vi "Application.vi"() -> ()   [LabVIEW 2021]
doc: "Application that demonstrates connecting to a DAQ device and activates the selected digital inputs and analog inputs. Stream the data from devices, logging the datapoints to CSV file and 2 plots."
uses:
  TypeDefs/TypeDef - Cluster of DAQiFi Device Properties.ctl
  TypeDefs/Enum - Connection Type.ctl
  <vilib>/Utility/file.llb/Write Delimited Spreadsheet (string).vi
  <vilib>/JDP Science/JDP Science Common Utilities/Timestamp/JDP Timestamp.lvlib
panel:
  in  "Data Logging Rate (Hz)":i32=10 min=1 max=1000 step=1
  in  "Start Logging":bool
  in  "Filepath to Save Data to (CSV)":path
  in  "Digital Channels":bool[](array[boolean])
  in  "Analog Channels":bool[](array[boolean])
  in  "Connect USB":bool
  out "Busy":u16(ring)
  out "Status":string
  in  "Connect WIFI":bool
  in  "Search USB":bool
  in  "Search WIFI":bool
  in  "DAQiFi Available USB Connections":i32(listbox)
  in  "DAQiFi Available Wireless Connections":i32(listbox)
  out "Digital Chart":T1(graph)
  out "Analog Chart":T2(graph)
  in  "stop":bool
  # "Enabled selected channels by left clicking the green boxes"
  # "0       1      2      3     4      5     6      7      8     9     10    11    12    13   14    15"
  # "0       1      2      3     4      5     6      7      8     9     10    11    12    13   14    15"
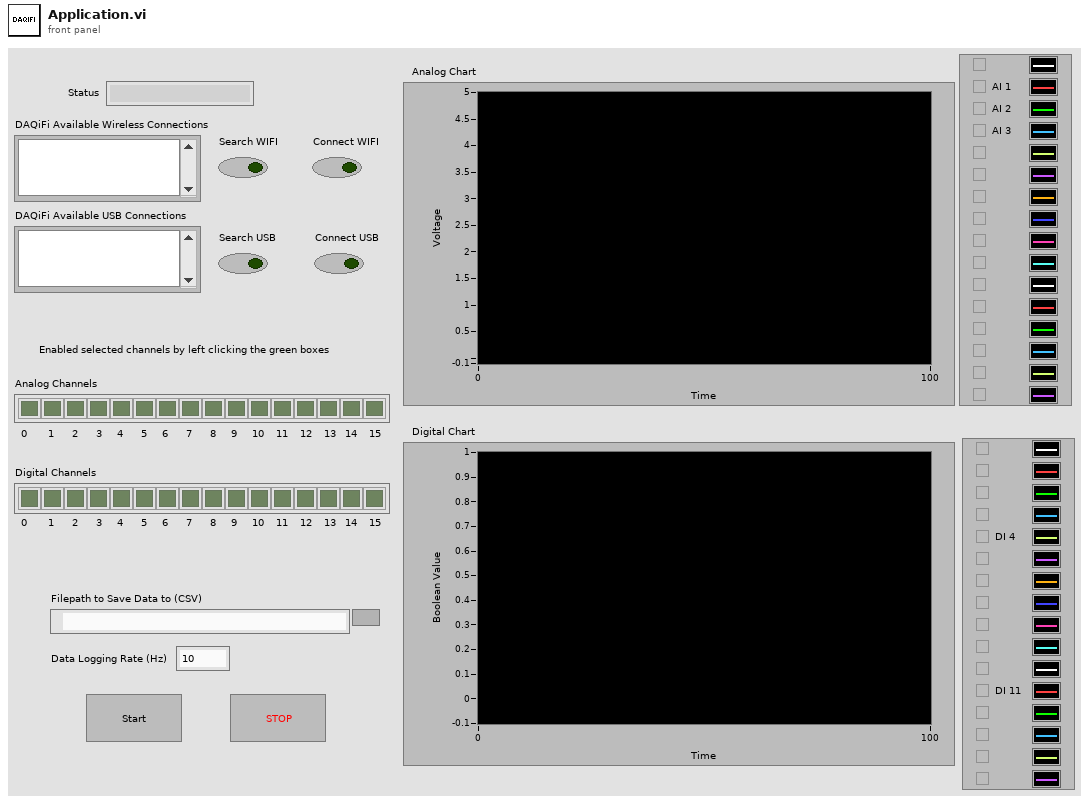
[diagram p1: front panel]
types:
  T1 = cluster{"[0]":dbl, "[1]":dbl, "[2]":dbl, "[3]":dbl, "[4]":dbl, "[5]":dbl, "[6]":dbl, "[7]":dbl, "[8]":dbl}
  T2 = cluster{"Array of Voltages (V)[0]":dbl, "Array of Voltages (V)[1]":dbl, "Array of Voltages (V)[2]":dbl, "Array of Voltages (V)[3]":dbl, "Array of Voltages (V)[4]":dbl, "Array of Voltages (V)[5]":dbl, "Array of Voltages (V)[6]":dbl, "Array of Voltages (V)[7]":dbl, "Array of Voltages (V)[8]":dbl}
  T3 = typedef "TypeDef - Cluster of DAQiFi Device Properties.ctl" = cluster{"IP Address":string, "MAC Address":string, "Serial Number":string, "Connection Type":T4, "Connected":bool, "TCP Network Connection":refnum<k5>, "USB Serial Connection":refnum<visa-resource-name>}
  T4 = typedef "Enum - Connection Type.ctl" = enum16{"USB", "TCP"}
  T5 = cluster{"Array of Voltages (V)[0]":dbl, "Array of Voltages (V)[1]":dbl, "Array of Voltages (V)[2]":dbl, "Array of Voltages (V)[3]":dbl, "Array of Voltages (V)[4]":dbl, "Array of Voltages (V)[5]":dbl, "Array of Voltages (V)[6]":dbl, "Array of Voltages (V)[7]":dbl, "Array of Voltages (V)[8]":dbl}[]
  T6 = enum8{"Enabled", "Disabled", "Disabled and Grayed Out"}
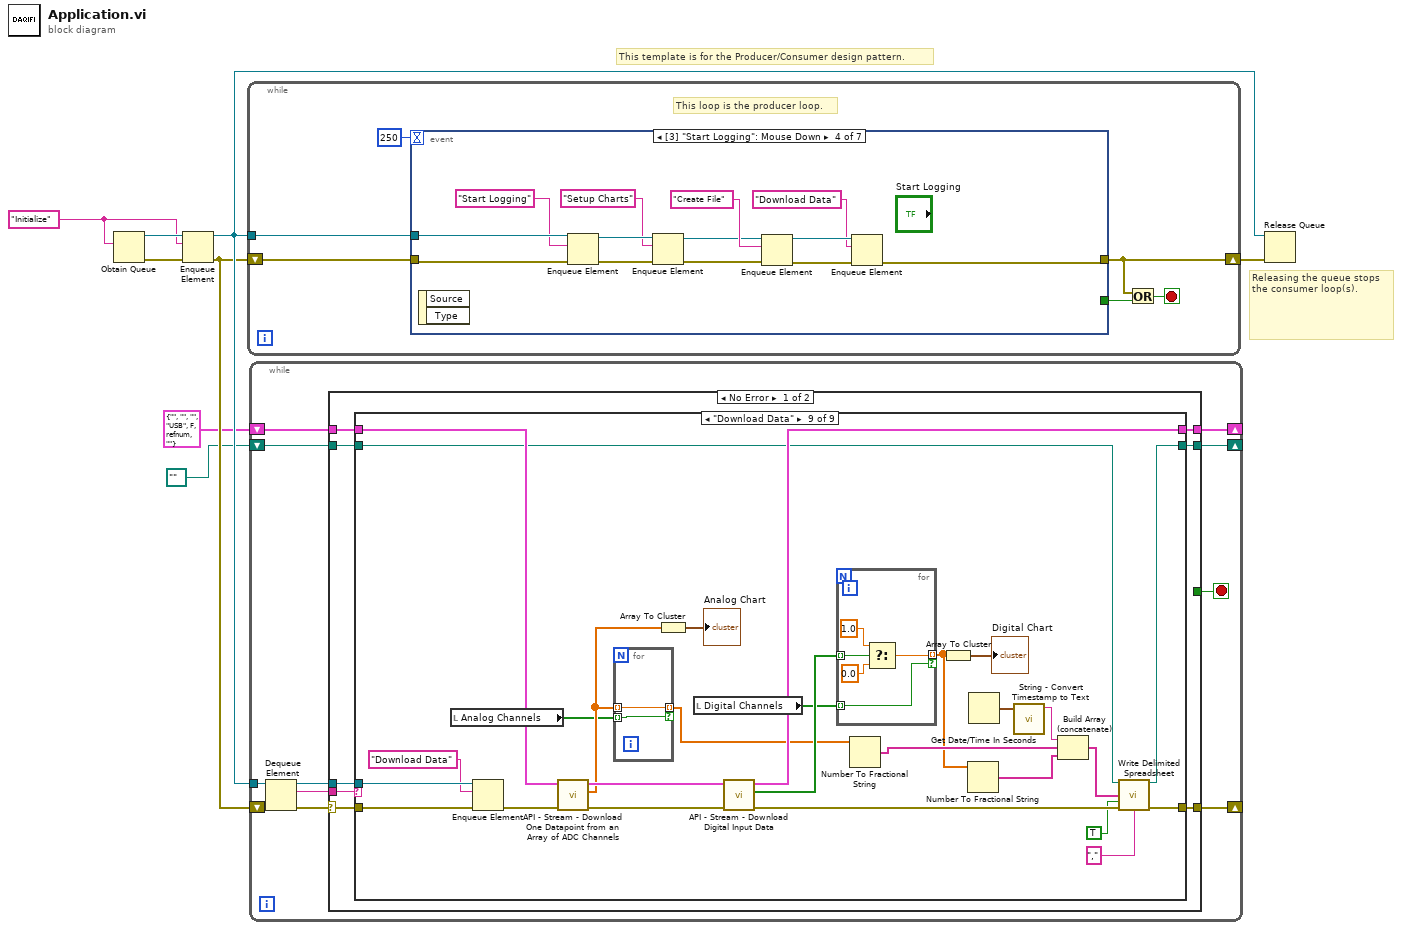
[diagram p0: block diagram]
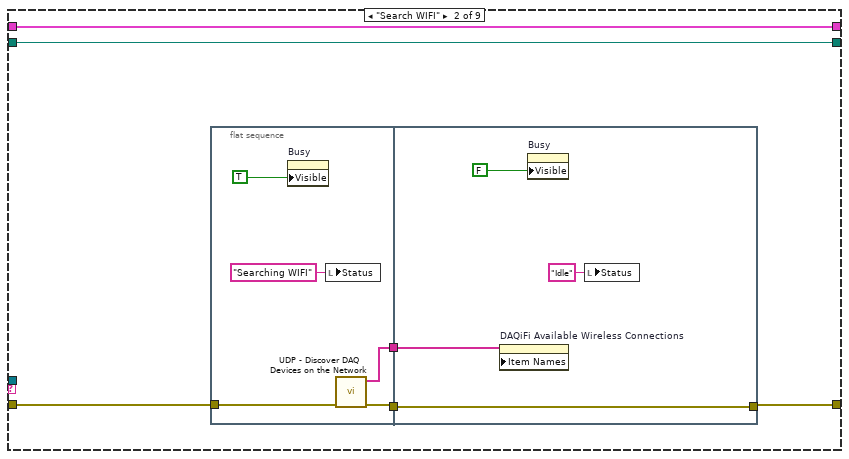
[diagram p3: hidden frame]
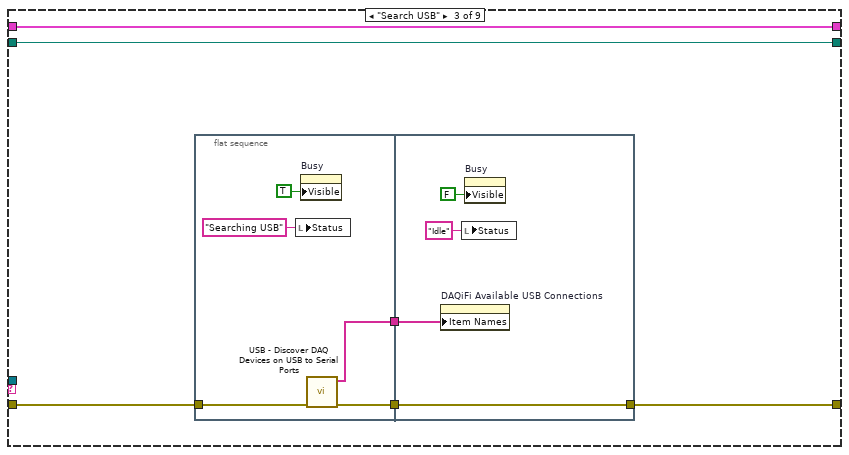
[diagram p4: hidden frame]
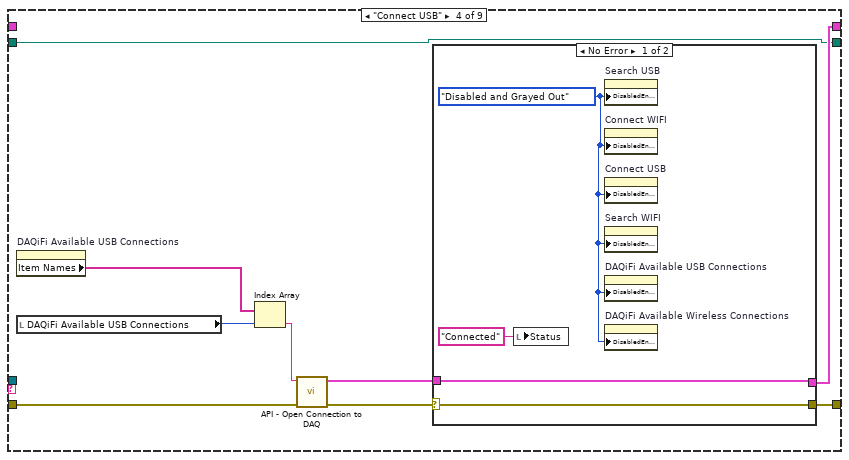
[diagram p5: hidden frame]
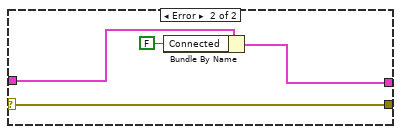
[diagram p6: hidden frame]
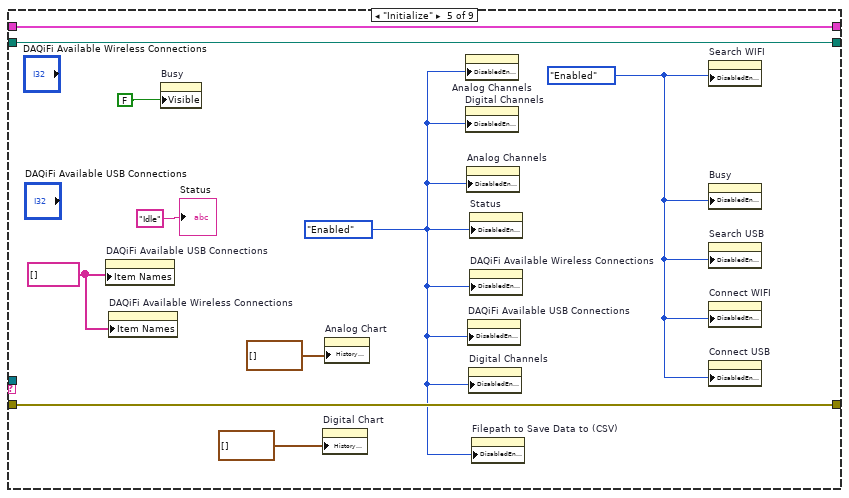
[diagram p7: hidden frame]
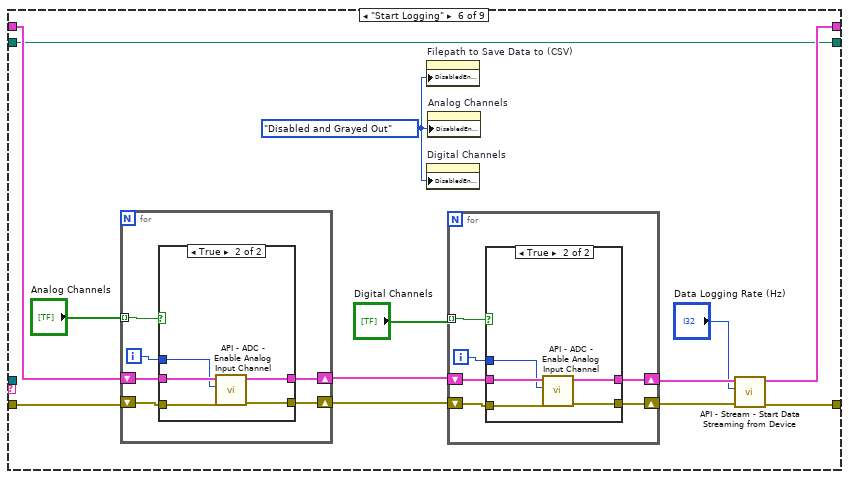
[diagram p8: hidden frame]
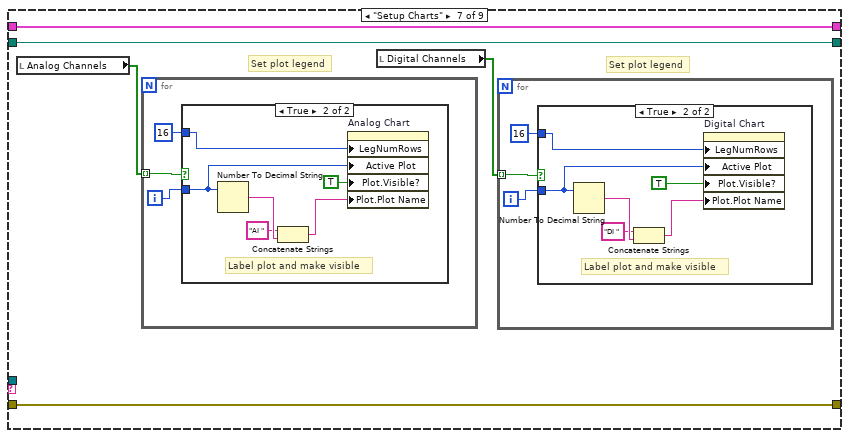
[diagram p11: hidden frame]
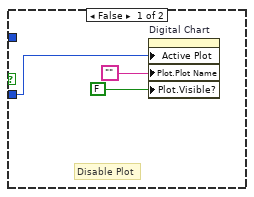
[diagram p12: hidden frame]
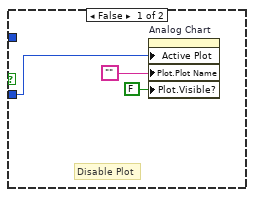
[diagram p13: hidden frame]
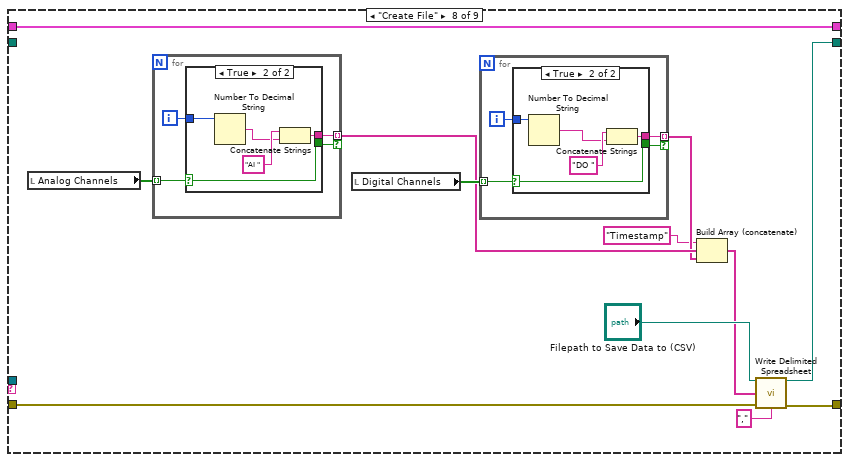
[diagram p14: hidden frame]
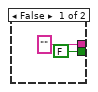
[diagram p15: hidden frame]
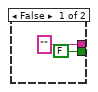
[diagram p16: hidden frame]
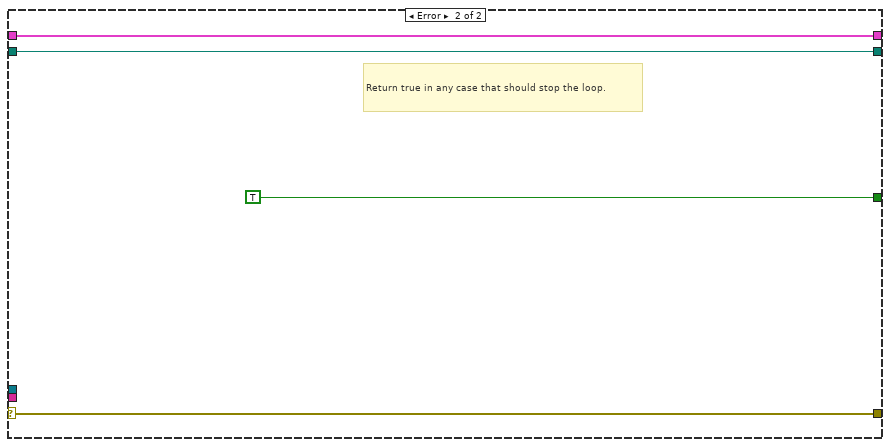
[diagram p17: hidden frame]
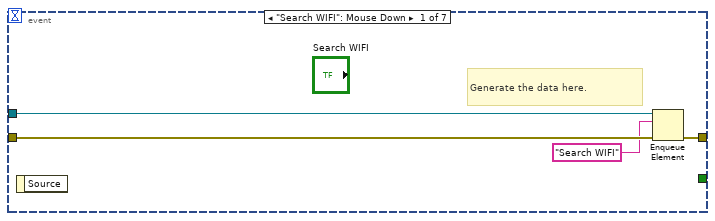
[diagram p18: hidden frame]
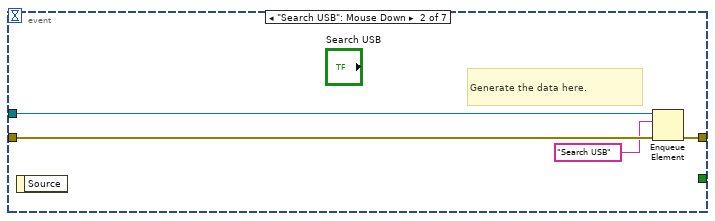
[diagram p19: hidden frame]
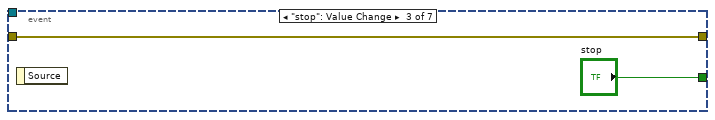
[diagram p20: hidden frame]
diagram:
  w4 = "Initialize"
  # "Releasing the queue stops the consumer loop(s)."
  # "This template is for the Producer/Consumer design pattern."
  n1 = Obtain Queue(element data type=w4) -> (queue out=w7:refnum<queue>, error out=w6:errorcluster)  [unwired: 4 in, 1 out]
  n2 = Enqueue Element(queue=w7, element=w4, error in (no error)=w6) -> (queue out=w5:refnum<queue>, error out=w3:errorcluster)  [unwired: 1 in, 1 out]
  n3 = while {
    shift-right: [w10] -> w8
    shift-left: w3 -> [w13]
    tunnel: w5 -> [w14]
    stop <- w11 stop-if-true
    # "This loop is the producer loop."
    n4 = event shown="[3] \"Start Logging\": Mouse Down" {
      selector: _ -> [_ _ _ _ _ _ _]
      dyn-events: _ -> [_ _ _ _ _ _ _]
      timeout: 250 -> [_ _ _ _ _ _ _]
      tunnel: w14 -> [w18 w22 _ w37 _ w47 w51]
      tunnel: w13 -> [w17 w21 w23 w36 _ w46 w50]
      tunnel: [w16 w20 w23 w33 _ w45 w49] -> w10
      tunnel: [_ _ "stop" _ _ _ _] -> w12
      event "Search WIFI": Mouse Down {
        # "Generate the data here."
        n5 = event-data() -> ()  [unwired: 1 in, 1 out]
        n6 = Enqueue Element(queue=w18, element="Search WIFI", error in (no error)=w17) -> (error out=w16:errorcluster)  [unwired: 1 in, 2 out]
      }
      event "Search USB": Mouse Down {
        # "Generate the data here."
        n7 = event-data() -> ()  [unwired: 1 in, 1 out]
        n8 = Enqueue Element(queue=w22, element="Search USB", error in (no error)=w21) -> (error out=w20:errorcluster)  [unwired: 1 in, 2 out]
      }
      event "stop": Value Change {
        n9 = event-data() -> ()  [unwired: 1 in, 1 out]
      }
      event "Start Logging": Mouse Down {
        n10 = event-data() -> ()  [unwired: 1 in, 2 out]
        n11 = Enqueue Element(queue=w37, element="Start Logging", error in (no error)=w36) -> (queue out=w26:refnum<queue>, error out=w29:errorcluster)  [unwired: 1 in, 1 out]
        n12 = Enqueue Element(queue=w26, element="Setup Charts", error in (no error)=w29) -> (queue out=w27:refnum<queue>, error out=w28:errorcluster)  [unwired: 1 in, 1 out]
        n13 = Enqueue Element(queue=w27, element="Create File", error in (no error)=w28) -> (queue out=w32:refnum<queue>, error out=w34:errorcluster)  [unwired: 1 in, 1 out]
        n14 = Enqueue Element(queue=w32, element="Download Data", error in (no error)=w34) -> (error out=w33:errorcluster)  [unwired: 1 in, 2 out]
      }
      event Timeout {
        n15 = event-data() -> ()  [unwired: 1 in, 2 out]
        n16 = local read "Busy"() -> (w43:u16)
        n17 = Increment(x=w43) -> (x+1=w39:u16)
        n18 = Greater?(x=w39, y=u16 6) -> (0:w41:bool)
        n19 = Select(t=u16 0, s=w41, f=w39) -> (s? t:f=→"Busy":u16)
      }
      event "Connect USB": Value Change {
        n20 = event-data() -> ()  [unwired: 1 in, 2 out]
        n21 = Enqueue Element(queue=w47, element="Connect USB", error in (no error)=w46) -> (error out=w45:errorcluster)  [unwired: 1 in, 2 out]
      }
      event "Connect WIFI": Value Change {
        n22 = event-data() -> ()  [unwired: 1 in, 2 out]
        n23 = Enqueue Element(queue=w51, element="Connect WIFI", error in (no error)=w50) -> (error out=w49:errorcluster)  [unwired: 1 in, 2 out]
      }
    }
    n24 = Or(x=w10, y=w12) -> (x .or. y?=w11:bool)
  }
  n25 = while {
    tunnel: w5 -> [w62]
    shift-right: [w58] -> _
    shift-left: w3 -> [w57]
    shift-right: [w56] -> _
    shift-left: T3 {"IP Address"="", "MAC Address"="", "Serial Number"="", "Connection Type"=enum."USB", "Connected"=FALSE, "TCP Network Connection"=refnum, "USB Serial Connection"=""} ("DAQiFi Device Properties") -> [w55]
    shift-right: [w54] -> _
    shift-left: path "" ("new file path (Not A Path if cancelled)") -> [w53]
    stop <- w59 stop-if-true
    n26 = Dequeue Element(queue=w62, error in (no error)=w57) -> (queue out=w52:refnum<queue>, element=w60:string, error out=w61:errorcluster)  [unwired: 1 in, 1 out]
    n27 = case shown="No Error" w61 {
      selector: w61 -> [w69 w268]
      tunnel: w60 -> [w70 _]
      tunnel: [_ TRUE] -> w59
      tunnel: [w68 w268] -> w58
      tunnel: [w67 w269] -> w56
      tunnel: w55 -> [w66 w269]
      tunnel: [w65 w267] -> w54
      tunnel: w53 -> [w64 w267]
      tunnel: w52 -> [w63 _]
      frame No Error {
        n28 = case shown="\"Download Data\"" w70 {
          tunnel: w69 -> [w73 w77 w93 w110 w129 w141 w174 w209 w258]
          tunnel: [w73 w75 w92 w105 w129 w135 w174 w208 w246] -> w68
          tunnel: [w72 w78 w94 w106 w128 w134 w173 w210 w252] -> w67
          tunnel: w66 -> [w72 w78 w94 _ w128 w142 w173 w210 w255]
          tunnel: [w71 w74 w89 w104 w123 w131 w172 w200 w244] -> w65
          tunnel: w64 -> [w71 w74 w89 w104 w123 w131 w172 _ w245]
          tunnel: w63 -> [_ _ _ _ _ _ _ _ w259]
          frame "False", Default {
          }
          frame "Search WIFI" {
            n29 = flat-sequence {
              tunnel: [w84] -> w79
              tunnel: w77 -> [w81]
              tunnel: [w80] -> w76
              tunnel: w79 -> [w88]
              tunnel: [w85] -> w75
              tunnel: w76 -> [w85]
              frame #0 {
                n30 = property on="Busy" class="Ring (strict)"("Visible"=TRUE) -> ()  [unwired: 2 in, 2 out]
                n31 = local write "Status"("Searching WIFI" ("Status")) -> ()
                n32 = call "UDP - Discover DAQ Devices on the Network.vi"("error in"=w81) -> ("Error out"=w80:errorcluster, "List of IPs"=w84:string[])  [unwired: 8 in, 1 out]
              }
              frame #1 {
                n33 = property on="DAQiFi Available Wireless Connections" class="LstBox (strict)"("Item Names"=w88) -> ()  [unwired: 2 in, 2 out]
                n34 = property on="Busy" class="Ring (strict)"("Visible"=FALSE) -> ()  [unwired: 2 in, 2 out]
                n35 = local write "Status"("Idle" ("Status")) -> ()
              }
            }
          }
          frame "Search USB" {
            n36 = flat-sequence {
              tunnel: w93 -> [w99]
              tunnel: [w98] -> w91
              tunnel: [w95] -> w90
              tunnel: [w103] -> w92
              tunnel: w91 -> [w103]
              tunnel: w90 -> [w100]
              frame #0 {
                n37 = local write "Status"("Searching USB" ("Status")) -> ()
                n38 = property on="Busy" class="Ring (strict)"("Visible"=TRUE) -> ()  [unwired: 2 in, 2 out]
                n39 = call "USB - Discover DAQ Devices on USB to Serial Ports.vi"("error in"=w99) -> ("error out"=w98:errorcluster, "List of DAQiFi COM Ports"=w95:string[])  [unwired: 8 in, 1 out]
              }
              frame #1 {
                n40 = property on="DAQiFi Available USB Connections" class="LstBox (strict)"("Item Names"=w100) -> ()  [unwired: 2 in, 2 out]
                n41 = local write "Status"("Idle" ("Status")) -> ()
                n42 = property on="Busy" class="Ring (strict)"("Visible"=FALSE) -> ()  [unwired: 2 in, 2 out]
              }
            }
          }
          frame "Connect USB" {
            n43 = property on="DAQiFi Available USB Connections" class="LstBox (strict)"() -> ("Item Names"=w112:string[])  [unwired: 2 in, 2 out]
            n44 = local read "DAQiFi Available USB Connections"() -> (w109:i32)
            n45 = Index Array(array=w112, index=w109) -> (element=w111:string)
            n46 = call "API - Open Connection to DAQ.vi"("error in"=w110, "DAQ Address (IP or COM)"=w111) -> ("error out"=w108:errorcluster, "DAQiFi Device Properties"=w107:T3)  [unwired: 8 in]
            n47 = case shown="No Error" w108 {
              selector: w108 -> [w116 w117]
              tunnel: w107 -> [w115 w120]
              tunnel: [w115 w118] -> w106
              tunnel: [w116 w117] -> w105
              frame No Error {
                w114 = T6."Disabled and Grayed Out" ("Disabled")
                n48 = local write "Status"("Connected" ("Status")) -> ()
                n49 = property on="Search USB" class="Bool (strict)"("DisabledEnum"=w114) -> ()  [unwired: 2 in, 2 out]
                n50 = property on="Connect WIFI" class="Bool (strict)"("DisabledEnum"=w114) -> ()  [unwired: 2 in, 2 out]
                n51 = property on="Connect USB" class="Bool (strict)"("DisabledEnum"=w114) -> ()  [unwired: 2 in, 2 out]
                n52 = property on="Search WIFI" class="Bool (strict)"("DisabledEnum"=w114) -> ()  [unwired: 2 in, 2 out]
                n53 = property on="DAQiFi Available USB Connections" class="LstBox (strict)"("DisabledEnum"=w114) -> ()  [unwired: 2 in, 2 out]
                n54 = property on="DAQiFi Available Wireless Connections" class="LstBox (strict)"("DisabledEnum"=w114) -> ()  [unwired: 2 in, 2 out]
              }
              frame Error {
                n55 = Bundle By Name(cluster=w120, "Connected"=FALSE) -> (w118:T3)
              }
            }
          }
          frame "Initialize" {
            w124 = T6."Enabled" ("Disabled")
            w125 = T6."Enabled" ("Disabled")
            w126 = string[] [] ("Item Names")
            n56 = property on="DAQiFi Available USB Connections" class="LstBox (strict)"("Item Names"=w126) -> ()  [unwired: 2 in, 2 out]
            n57 = property on="DAQiFi Available Wireless Connections" class="LstBox (strict)"("Item Names"=w126) -> ()  [unwired: 2 in, 2 out]
            n58 = property on="Busy" class="Ring (strict)"("Visible"=FALSE) -> ()  [unwired: 2 in, 2 out]
            n59 = property on="Digital Chart" class="WFChart (strict)"("History Data"=T5 []) -> ()  [unwired: 2 in, 2 out]
            n60 = property on="Analog Chart" class="WFChart (strict)"("History Data"=T5 []) -> ()  [unwired: 2 in, 2 out]
            n61 = property on="Analog Channels" class="Arr (strict)"("DisabledEnum"=w124) -> ()  [unwired: 2 in, 2 out]
            n62 = property on="Digital Channels" class="Arr (strict)"("DisabledEnum"=w124) -> ()  [unwired: 2 in, 2 out]
            n63 = property on="Analog Channels" class="Arr (strict)"("DisabledEnum"=w124) -> ()  [unwired: 2 in, 2 out]
            n64 = property on="DAQiFi Available USB Connections" class="LstBox (strict)"("DisabledEnum"=w124) -> ()  [unwired: 2 in, 2 out]
            n65 = property on="Digital Channels" class="Arr (strict)"("DisabledEnum"=w124) -> ()  [unwired: 2 in, 2 out]
            n66 = property on="Status" class="Str"("DisabledEnum"=w124) -> ()  [unwired: 2 in, 2 out]
            n67 = property on="DAQiFi Available Wireless Connections" class="LstBox (strict)"("DisabledEnum"=w124) -> ()  [unwired: 2 in, 2 out]
            n68 = property on="Filepath to Save Data to (CSV)" class="Path"("DisabledEnum"=w124) -> ()  [unwired: 2 in, 2 out]
            n69 = property on="Search WIFI" class="Bool (strict)"("DisabledEnum"=w125) -> ()  [unwired: 2 in, 2 out]
            n70 = property on="Busy" class="Ring (strict)"("DisabledEnum"=w125) -> ()  [unwired: 2 in, 2 out]
            n71 = property on="Search USB" class="Bool (strict)"("DisabledEnum"=w125) -> ()  [unwired: 2 in, 2 out]
            n72 = property on="Connect WIFI" class="Bool (strict)"("DisabledEnum"=w125) -> ()  [unwired: 2 in, 2 out]
            n73 = property on="Connect USB" class="Bool (strict)"("DisabledEnum"=w125) -> ()  [unwired: 2 in, 2 out]
            "Status" <- "Idle" ("Status")
          }
          frame "Start Logging" {
            w132 = T6."Disabled and Grayed Out" ("Disabled")
            n74 = for {
              tunnel: "Analog Channels" -> [w161] mode=indexing
              shift-right: [w158] -> w139
              shift-left: w142 -> [w162]
              shift-right: [w159] -> w138
              shift-left: w141 -> [w160]
              i -> [w157]
              n75 = case shown="True" w161 {
                tunnel: w162 -> [w164 w169]
                tunnel: w160 -> [w163 w168]
                tunnel: [w163 w167] -> w159
                tunnel: [w164 w166] -> w158
                tunnel: w157 -> [_ w165]
                frame False {
                }
                frame True {
                  n76 = call "API - ADC - Enable Analog Input Channel.vi"("error in (no error)"=w168, "Analog Input Channel Number"=w165, "DAQiFi Device Properties In"=w169) -> ("error out"=w167:errorcluster, "DAQiFi Device Properties Out"=w166:T3)  [unwired: 7 in]
                }
              }
            }
            n77 = property on="Filepath to Save Data to (CSV)" class="Path"("DisabledEnum"=w132) -> ()  [unwired: 2 in, 2 out]
            n78 = property on="Digital Channels" class="Arr (strict)"("DisabledEnum"=w132) -> ()  [unwired: 2 in, 2 out]
            n79 = property on="Analog Channels" class="Arr (strict)"("DisabledEnum"=w132) -> ()  [unwired: 2 in, 2 out]
            n80 = for {
              tunnel: "Digital Channels" -> [w148] mode=indexing
              shift-right: [w145] -> w136
              shift-left: w139 -> [w149]
              shift-right: [w146] -> w137
              shift-left: w138 -> [w147]
              i -> [w144]
              n81 = case shown="True" w148 {
                tunnel: w149 -> [w151 w156]
                tunnel: w147 -> [w150 w155]
                tunnel: [w150 w154] -> w146
                tunnel: [w151 w153] -> w145
                tunnel: w144 -> [_ w152]
                frame False {
                }
                frame True {
                  n82 = call "API - ADC - Enable Analog Input Channel.vi"("error in (no error)"=w155, "Analog Input Channel Number"=w152, "DAQiFi Device Properties In"=w156) -> ("error out"=w154:errorcluster, "DAQiFi Device Properties Out"=w153:T3)  [unwired: 7 in]
                }
              }
            }
            n83 = call "API - Stream - Start Data Streaming from Device.vi"("error in"=w137, "Streaming Rate (Hz)"="Data Logging Rate (Hz)", "DAQiFi Device Properties In"=w136) -> ("error out"=w135:errorcluster, "DAQiFi Device Properties Out"=w134:T3)  [unwired: 7 in]
          }
          frame "Setup Charts" {
            # "Set plot legend"
            # "Set plot legend"
            n84 = local read "Analog Channels"() -> (w171:bool[])
            n85 = for {
              tunnel: w171 -> [w189] mode=indexing
              i -> [w188]
              n86 = case shown="True" w189 {
                tunnel: w188 -> [w190 w194]
                tunnel: 16 -> [_ w193]
                frame False {
                  # "Disable Plot"
                  n87 = property on="Analog Chart" class="WFChart (strict)"("Active Plot"=w190, "Plot.Plot Name"="", "Plot.Visible?"=FALSE ("Plot.Visible")) -> ()  [unwired: 2 in, 2 out]
                }
                frame True {
                  # "Label plot and make visible"
                  n88 = Number To Decimal String(number=w194) -> (decimal integer string=w197:string)  [unwired: 1 in]
                  n89 = Concatenate Strings("AI " ("string"), w197) -> (w195:string)
                  n90 = property on="Analog Chart" class="WFChart (strict)"("LegNumRows"=w193, "Active Plot"=w194, "Plot.Visible?"=TRUE ("Plot.Visible"), "Plot.Plot Name"=w195) -> ()  [unwired: 2 in, 2 out]
                }
              }
            }
            n91 = local read "Digital Channels"() -> (w170:bool[])
            n92 = for {
              tunnel: w170 -> [w177] mode=indexing
              i -> [w176]
              n93 = case shown="True" w177 {
                tunnel: w176 -> [w178 w182]
                tunnel: 16 -> [_ w181]
                frame False {
                  # "Disable Plot"
                  n94 = property on="Digital Chart" class="WFChart (strict)"("Active Plot"=w178, "Plot.Plot Name"="", "Plot.Visible?"=FALSE ("Plot.Visible")) -> ()  [unwired: 2 in, 2 out]
                }
                frame True {
                  # "Label plot and make visible"
                  n95 = Number To Decimal String(number=w182) -> (decimal integer string=w185:string)  [unwired: 1 in]
                  n96 = Concatenate Strings("DI " ("string"), w185) -> (w183:string)
                  n97 = property on="Digital Chart" class="WFChart (strict)"("LegNumRows"=w181, "Active Plot"=w182, "Plot.Visible?"=TRUE ("Plot.Visible"), "Plot.Plot Name"=w183) -> ()  [unwired: 2 in, 2 out]
                }
              }
            }
          }
          frame "Create File" {
            n98 = local read "Analog Channels"() -> (w205:bool[])
            n99 = for {
              tunnel: w205 -> [w225] mode=indexing
              tunnel: [w223] -> w203 mode=indexing if=w222
              i -> [w224]
              n100 = case shown="True" w225 {
                selector: w225 -> [_ w230]
                tunnel: w224 -> [_ w232]
                tunnel: ["" w231] -> w223
                tunnel: [FALSE w230] -> w222
                frame False {
                }
                frame True {
                  n101 = Number To Decimal String(number=w232) -> (decimal integer string=w228:string)  [unwired: 1 in]
                  n102 = Concatenate Strings("AI ", w228) -> (w231:string)
                }
              }
            }
            n103 = local read "Digital Channels"() -> (w204:bool[])
            n104 = for {
              tunnel: w204 -> [w214] mode=indexing
              tunnel: [w212] -> w202 mode=indexing if=w211
              i -> [w213]
              n105 = case shown="True" w214 {
                selector: w214 -> [_ w219]
                tunnel: w213 -> [_ w221]
                tunnel: ["" w220] -> w212
                tunnel: [FALSE w219] -> w211
                frame False {
                }
                frame True {
                  n106 = Number To Decimal String(number=w221) -> (decimal integer string=w217:string)  [unwired: 1 in]
                  n107 = Concatenate Strings("DO ", w217) -> (w220:string)
                }
              }
            }
            n108 = Build Array (concatenate)("Timestamp", w203, w202) -> (w201:string[])
            n109 = call-poly <vilib>:"Write Delimited Spreadsheet.vi"("file path (dialog if empty)"="Filepath to Save Data to (CSV)", "1D data"=w201, "error in (no error)"=w209, "delimiter (\\t)"="," ("delimiter (\\t)")) -> ("new file path (Not A Path if cancelled)"=w200:path, "error out"=w208:errorcluster)  [unwired: 10 in]
          }
          frame "Download Data" {
            n110 = local read "Analog Channels"() -> (w234:bool[])
            n111 = Enqueue Element(queue=w259, element="Download Data", error in (no error)=w258) -> (error out=w256:errorcluster)  [unwired: 1 in, 2 out]
            n112 = call "API - Stream - Download One Datapoint from an Array of ADC Channels.vi"("error in"=w256, "DAQiFi Device Properties In"=w255) -> ("error out"=w253:errorcluster, "Array of Voltages (V)"=w235:dbl[], "DAQiFi Device Properties Out"=w254:T3)  [unwired: 7 in]
            n113 = for {
              tunnel: w235 -> [w261] mode=indexing
              tunnel: [w261] -> w233 mode=indexing if=w260
              tunnel: w234 -> [w260] mode=indexing
            }
            n114 = Array To Cluster(array=w235) -> (cluster=→"Analog Chart":T2)
            n115 = local read "Digital Channels"() -> (w250:bool[])
            n116 = call "API - Stream - Download Digital Input Data.vi"("error in"=w253, "DAQiFi Device Properties In"=w254) -> ("error out"=w247:errorcluster, "Digital Inputs"=w251:bool[], "DAQiFi Device Properties Out"=w252:T3)  [unwired: 7 in]
            n117 = for {
              tunnel: w251 -> [w266] mode=indexing
              tunnel: [w263] -> w240 mode=indexing if=w262
              tunnel: w250 -> [w262] mode=indexing
              n118 = Select(t=1.0, s=w266, f=0.0) -> (s? t:f=w263:dbl)
            }
            n119 = Number To Fractional String(number=w233) -> (F-format string=w241:string[])  [unwired: 3 in]
            n120 = Array To Cluster(array=w240) -> (cluster=→"Digital Chart":T1)
            n121 = Number To Fractional String(number=w240) -> (F-format string=w239:string[])  [unwired: 3 in]
            n122 = Get Date/Time In Seconds() -> (seconds since 1Jan1904=w243:timestamp)
            n123 = call "String - Convert Timestamp to Text.vi"("Time Stamp"=w243) -> ("Timestamp (RFC3339)"=w242:string)  [unwired: 9 in, 1 out]
            n124 = Build Array (concatenate)(w242, w241, w239) -> (w238:string[])
            n125 = call-poly <vilib>:"Write Delimited Spreadsheet.vi"("file path (dialog if empty)"=w245, "1D data"=w238, "append to file? (new file:F)"=TRUE, "error in (no error)"=w247, "delimiter (\\t)"="," ("delimiter (\\t)")) -> ("new file path (Not A Path if cancelled)"=w244:path, "error out"=w246:errorcluster)  [unwired: 9 in]
          }
        }
      }
      frame Error {
        # "Return true in any case that should stop the loop."
      }
    }
  }
  n126 = Release Queue(queue=w5, error in (no error)=w8) -> ()  [unwired: 1 in, 3 out]
